vi "radiant.vi"(7 "override":bool, 8 "error in (no error)":errorcluster, 10 "WL (nm)":dbl=644.0 format="%#_16g", 11 "VISA IN":refnum<visa-resource-name>="COM9") -> (0 "error out":errorcluster, 2 "value out":dbl=644.0 format="%#_16p", 3 "VISA resource out":refnum<visa-resource-name>)   [LabVIEW 2017]
uses:
  hardware/radiant/radiant.lvlib
panel:
  in  "VISA (default)":refnum<visa-resource-name>="COM9"
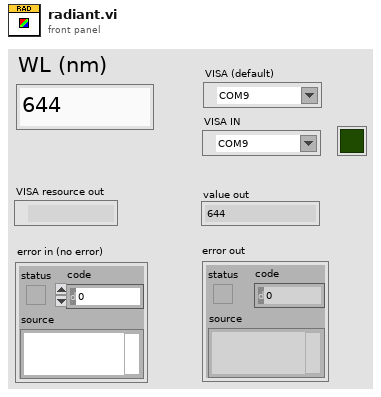
[diagram p1: front panel]
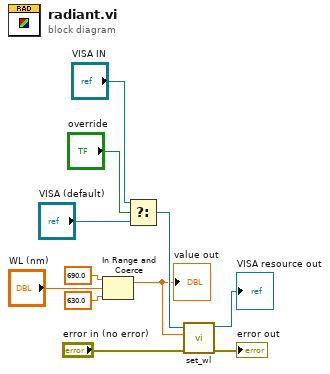
[diagram p0: block diagram]
diagram:
  n1 = In Range and Coerce(upper limit=690.0, x="WL (nm)", lower limit=630.0 ("x")) -> (coerced(x)=w3:dbl)  [unwired: 1 out]
  "value out" <- w3
  n2 = Select(t="VISA IN", s="override", f="VISA (default)") -> (s? t:f=w7:refnum<visa-resource-name>)
  n3 = call "set_wl.vi"("error in (no error)"="error in (no error)", "fundamental (nm)"=w3, "VISA resource name"=w7) -> ("error out"=→"error out":errorcluster, "VISA resource name out"=→"VISA resource out":refnum<visa-resource-name>)  [unwired: 6 in, 1 out]
